vi "Find Test Cases in Application Instance.vi"(8 "error in (no error)":errorcluster) -> (0 "error out":errorcluster, 1 "Classes in App Instance":string[](array[string]), 2 "Class Paths":path[](array[path]), 3 "Project Path":path)   [LabVIEW 2020, in "Test Finder.lvclass"]
uses:
  Test Finder.lvclass
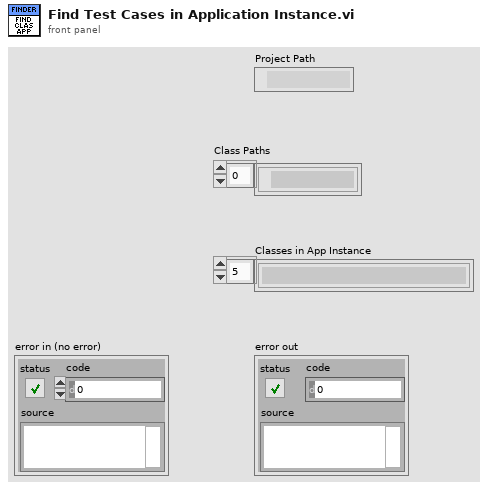
[diagram p1: front panel]
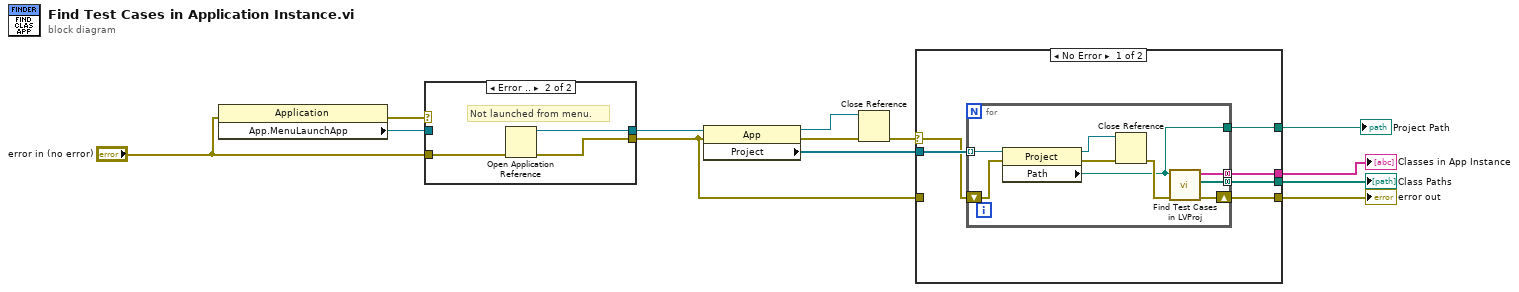
[diagram p0: block diagram]
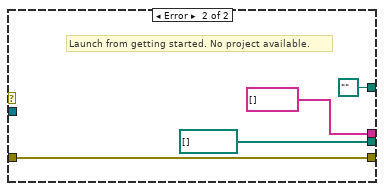
[diagram p2: hidden frame]
diagram:
  n1 = property class="Application"(error in="error in (no error)") -> (error out=w10:errorcluster, "App.MenuLaunchApp"=w9:refnum<vi>)  [unwired: 1 in, 1 out]
  n2 = case shown="Error .." w10 {
    selector: w10 -> [w14 _]
    tunnel: [w15 w18] -> w8
    tunnel: w9 -> [w15 _]
    tunnel: [w14 w17] -> w1
    tunnel: "error in (no error)" -> [_ w16]
    frame No Error {
      # "Launch from menu"
    }
    frame Error {
      # "Not launched from menu."
      n3 = Open Application Reference(8:w16) -> (0:w17:errorcluster, 3:w18:refnum<vi>)  [unwired: 3 in]
    }
  }
  n4 = property class="App"(reference=w8, error in=w1) -> (reference out=w13:refnum<vi>, error out=w12:errorcluster, "Project"=w11:refnum<vi>[])
  n5 = Close Reference(reference=w13, error in (no error)=w12) -> (error out=w7:errorcluster)
  n6 = case shown="No Error" w7 {
    selector: w7 -> [w23 _]
    tunnel: w11 -> [w24 _]
    tunnel: [w22 path[] [] ("Class paths")] -> w6
    tunnel: [w21 string[] [] ("Classes in project")] -> w5
    tunnel: [w20 w34] -> w4
    tunnel: [w19 path "" ("Path")] -> w3
    tunnel: w1 -> [_ w34]
    frame No Error {
      n7 = for {
        tunnel: w24 -> [w31] mode=indexing
        shift-right: [w29] -> w20
        shift-left: w23 -> [w28]
        tunnel: [w27] -> w22 mode=concatenating
        tunnel: [w26] -> w21 mode=concatenating
        tunnel: [w25] -> w19
        n8 = property class="Project"(reference=w31, error in=w28) -> (reference out=w33:refnum<vi>, error out=w32:errorcluster, "Path"=w25:path)
        n9 = Close Reference(reference=w33, error in (no error)=w32) -> (error out=w30:errorcluster)
        n10 = call "Find Test Cases in LVProj.vi"("error in (no error)"=w30, "Project Path"=w25) -> ("error out"=w29:errorcluster, "Class paths"=w27:path[], "Classes in project"=w26:string[])  [unwired: 7 in]
      }
    }
    frame Error {
      # "Launch from getting started. No project available."
    }
  }
  "error out" <- w4
  "Classes in App Instance" <- w5
  "Class Paths" <- w6
  "Project Path" <- w3
